vi "getMain.vi"(8 "error in (no error)":errorcluster, 11 "Theme.Colors in":refnum<class "Theme.Colors.lvclass">) -> (0 "error out":errorcluster, 2 "Main":T1={"Primary"=15224622, "Primary Variant"=16744512, "Secondary"=9342606, "Secondary Varient"=2039583}, 3 "Theme.Colors out":refnum<class "Theme.Colors.lvclass">)   [LabVIEW 2017, in "Theme.lvlib" / "Theme.Colors.lvclass"]
uses:
  Theme.Colors.lvclass
  Theme.Colors.lvclass/Theme.Colors.ctl
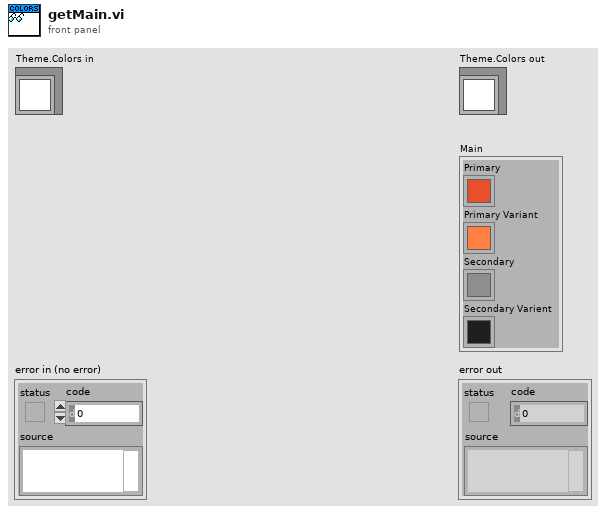
[diagram p1: front panel]
types:
  T1 = cluster{"Primary":u32, "Primary Variant":u32, "Secondary":u32, "Secondary Varient":u32}
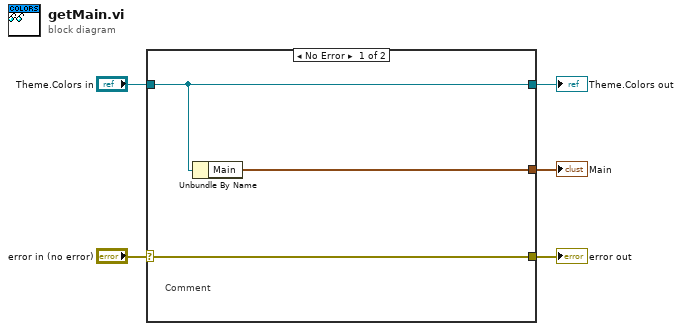
[diagram p0: block diagram]
diagram:
  n1 = case shown="No Error" "error in (no error)" {
    selector: "error in (no error)" -> [w8 w9]
    tunnel: [w8 w9] -> w4
    tunnel: [w7 w10] -> w2
    tunnel: "Theme.Colors in" -> [w7 w10]
    tunnel: [w6 _] -> w1
    frame No Error {
      # "Comment"
      n2 = Unbundle By Name(w7) -> ("Main"=w6:T1)
    }
    frame Error {
    }
  }
  "error out" <- w4
  "Theme.Colors out" <- w2
  "Main" <- w1
